vi "server.Parse Response (Object).vi"(8 "error in":errorcluster, 10 "Response String In":string) -> (0 "error out":errorcluster, 1 "LabVIEW Error?":bool=TRUE, 2 "JSON Array":refnum<class "JSON Object.lvclass">)   [LabVIEW 2016, in "JSONRPC Server.lvclass"]
uses:
  JSONRPC Server.lvclass
  <vilib>/NI/JSON Support for LabVIEW/JSON Data Classes/JSON Object/JSON Object.lvclass
  <vilib>/NI/JSON Support for LabVIEW/JSON Data Classes/JSON Helper/To More Specific Type (Object).vi
  <vilib>/NI/JSON Support for LabVIEW/JSON Data Classes/JSON Helper/JSON Helper.lvclass
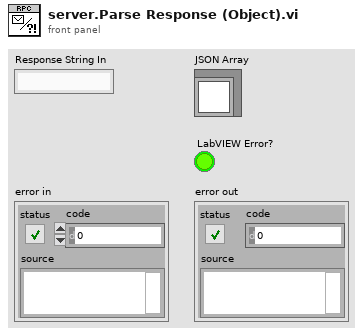
[diagram p1: front panel]
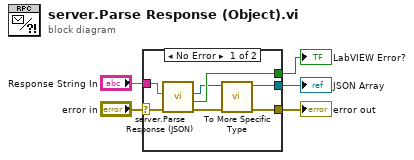
[diagram p0: block diagram]
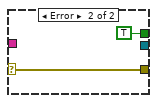
[diagram p2: hidden frame]
diagram:
  n1 = case shown="No Error" "error in" {
    selector: "error in" -> [w11 w14]
    tunnel: "Response String In" -> [w12 _]
    tunnel: [w10 TRUE ("LabVIEW Error?")] -> w3
    tunnel: [w7 w14] -> w2
    tunnel: [w6 _] -> w1
    frame No Error {
      n2 = call "server.Parse Response (JSON).vi"("error in"=w11, "Response String In"=w12) -> ("error out"=w8:errorcluster, "LabVIEW Error?"=w10:bool, "JSON out"=w9:refnum<class "JSON Null.lvclass">)  [unwired: 7 in]
      n3 = call-poly <vilib>:"To More Specific Type.vi"("error in (no error)"=w8, "JSON Datatype in"=w9) -> ("error out"=w7:errorcluster, "JSON Datatype out"=w6:refnum<class "JSON Object.lvclass">)  [unwired: 8 in]
    }
    frame Error {
    }
  }
  "error out" <- w2
  "LabVIEW Error?" <- w3
  "JSON Array" <- w1
